vi "Arduino_a.vi"(7 "Channel Number":i32, 8 "error in (no error)":errorcluster, 9 "Current  Setting":u8[](array[numeric]), 10 "Current Mode Count":i32, 11 "VISA Refnum in":refnum<visa-resource-name>) -> (0 "error out":errorcluster, 3 "VISA Refnum out":refnum<visa-resource-name>)   [LabVIEW 2023]
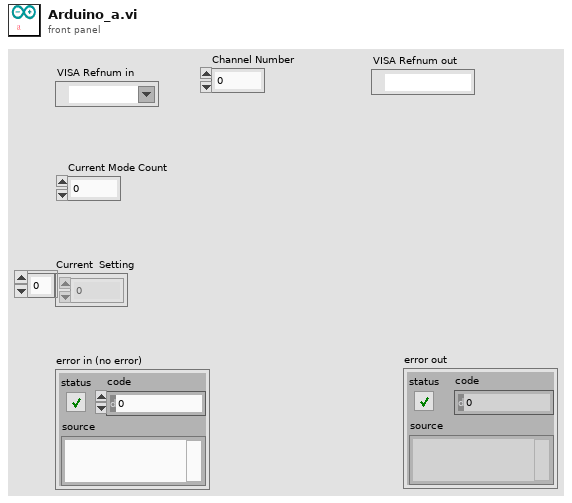
[diagram p1: front panel]
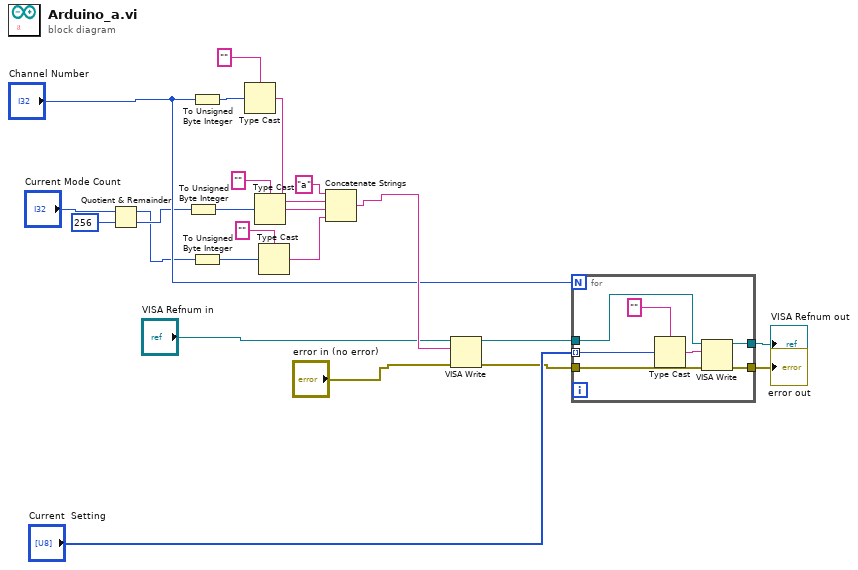
[diagram p0: block diagram]
diagram:
  n1 = Quotient & Remainder(x="Current Mode Count", y=256) -> (x-y*floor(x/y)=w2:i32, floor(x/y)=w3:i32)
  n2 = To Unsigned Byte Integer(number=w3) -> (unsigned 8bit integer=w20:u8)
  n3 = To Unsigned Byte Integer(number="Channel Number") -> (unsigned 8bit integer=w17:u8)
  n4 = To Unsigned Byte Integer(number=w2) -> (unsigned 8bit integer=w6:u8)
  n5 = Type Cast(type="" ("string"), x=w17) -> (*(type *) &x=w18:string)
  n6 = Type Cast(type="" ("string"), x=w20) -> (*(type *) &x=w19:string)
  n7 = Type Cast(type="" ("string"), x=w6) -> (*(type *) &x=w1:string)
  n8 = Concatenate Strings("a" ("data in"), w18, w19, w1) -> (w13:string)
  n9 = VISA Write(VISA resource name="VISA Refnum in", write buffer=w13, error in (no error)="error in (no error)") -> (VISA resource name out=w9:refnum<visa-resource-name>, error out=w10:errorcluster)  [unwired: 1 out]
  n10 = for {
    N: "Channel Number" -> [_]
    tunnel: "Current  Setting" -> [w25] mode=indexing
    tunnel: w10 -> [w30]
    tunnel: w9 -> [w29]
    tunnel: [w28] -> w15
    tunnel: [w27] -> w14
    n11 = Type Cast(type="" ("string"), x=w25) -> (*(type *) &x=w24:string)
    n12 = VISA Write(VISA resource name=w29, write buffer=w24, error in (no error)=w30) -> (VISA resource name out=w27:refnum<visa-resource-name>, error out=w28:errorcluster)  [unwired: 1 out]
  }
  "error out" <- w15
  "VISA Refnum out" <- w14
